vi "Revision Query.vi"(0 "VISA resource name":refnum<visa-resource-name>, 1 "Unit Address (1)":u8=1, 11 "error in (no error)":errorcluster {"code" format="%.0x"}) -> (4 "VISA resource name out":refnum<visa-resource-name>, 8 "Instr Driver Revision":string, 10 "Instr Firmware Revision":string, 15 "error out":errorcluster {"code" format="%.0x"})   [LabVIEW 2010]
doc: "This VI queries the current instrument firmware revision and instrument driver revision.\n\nThis Instrument Driver's Revision number is 1.0.0 and is compatible with Instrument Firmware Revision 7.00\n\nWLF4 Watlow Ramping Controller\nCreated By: Tomas Gres, VSB-TU Ostrava\nRelease Date: 03/2004\nOriginally Developed in LabVIEW Version: 6.1\n\nModification History: \n\nNone"
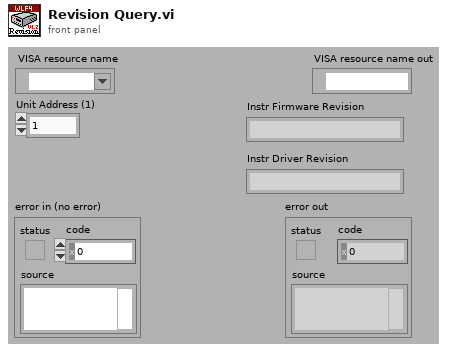
[diagram p1: front panel]
types:
  T1 = enum32{"invalid app kind", "Development System", "Run Time System", "Student Edition", "Embedded LabVIEW", "Evaluation", "Custom"}
  T2 = cluster{"Major":u16, "Minor":u16, "Fix":u16, "Build":u16}
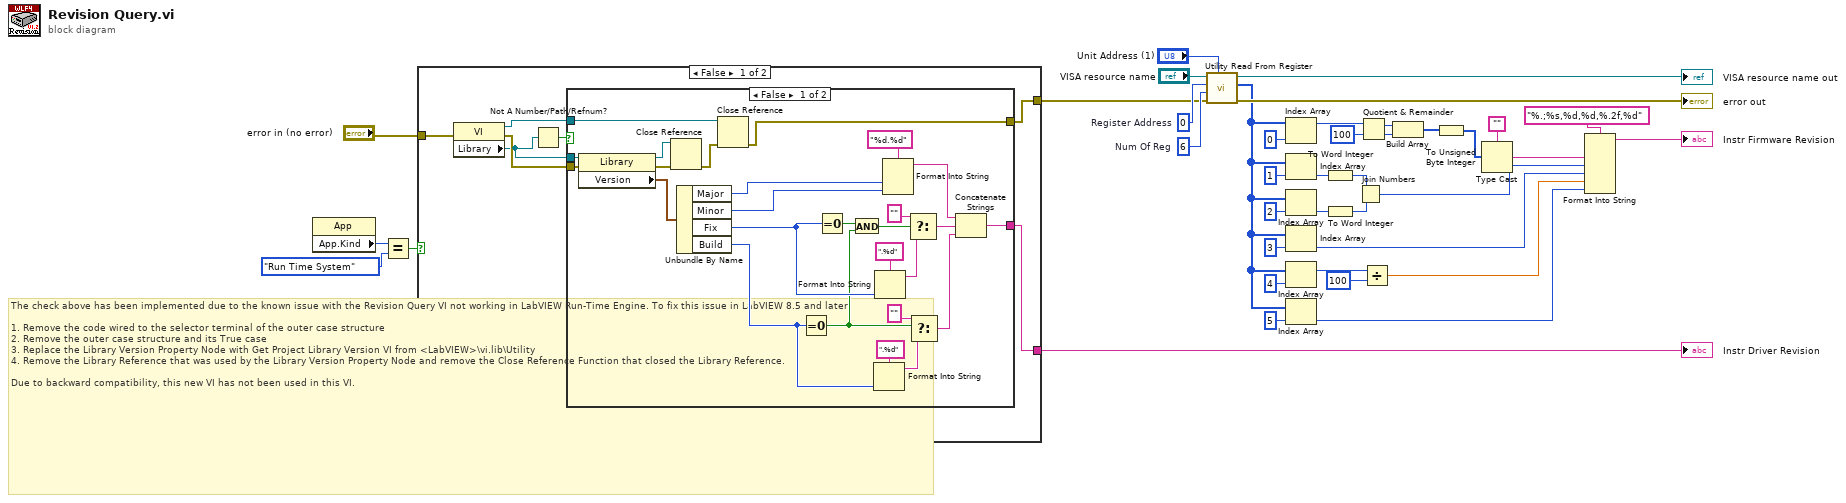
[diagram p0: block diagram]
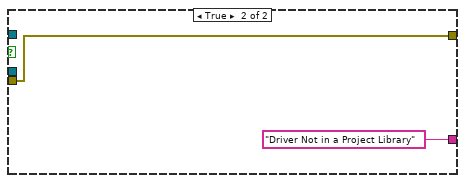
[diagram p2: hidden frame]
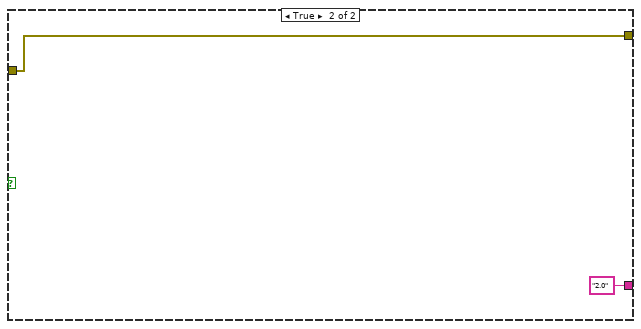
[diagram p3: hidden frame]
diagram:
  w34 = u16 6  # Num Of Reg
  w35 = u16 0  # Register Address
  # "The check above has been implemented due to the known issue with the Revision Query VI not working in LabVIEW Run-Time Engine. To fix this issue in LabVIEW 8.5 and later:\n\n1. Remove the code wired to the selector terminal of the outer case structure\n2. Remove the outer case structure and its True case\n3. Replace the Library Version Property Node with Get Project Library Version VI from <LabVIEW>\\vi.lib\\Utility\n4. Remove the Library Reference that was used by the Library Version Property Node and remove the Close Reference Function that closed the Library Reference.\n\nDue to backward compatibility, this new VI has not been used in this VI."
  n1 = property class="App"() -> ("App.Kind"=w3:T1)  [unwired: 2 in, 2 out]
  n2 = Equal?(x=w3, y=T1."Run Time System") -> (x = y?=w1:bool)
  n3 = case shown="False" w1 {
    tunnel: "error in (no error)" -> [w46 w76]
    tunnel: [w41 "2.0"] -> w5
    tunnel: [w40 w76] -> w4
    frame False {
      n4 = property class="VI"(error in=w46) -> (reference out=w42:refnum<vi>, error out=w45:errorcluster, "Library"=w44:refnum<vi>)  [unwired: 1 in]
      n5 = Not A Number/Path/Refnum?(number/path/refnum=w44) -> (NaN/Path/Refnum?=w43:bool)
      n6 = case shown="False" w43 {
        tunnel: [w51 w73] -> w40
        tunnel: [w50 "Driver Not in a Project Library"] -> w41
        tunnel: w45 -> [w49 w73]
        tunnel: w44 -> [w48 _]
        tunnel: w42 -> [w47 _]
        frame False {
          n7 = property class="Library"(reference=w48, error in=w49) -> (reference out=w71:refnum<vi>, error out=w72:errorcluster, "Version"=w69:T2)
          n8 = Close Reference(reference=w71, error in (no error)=w72) -> (error out=w70:errorcluster)
          n9 = Unbundle By Name(w69) -> ("Major"=w58:u16, "Minor"=w57:u16, "Fix"=w55:u16, "Build"=w56:u16)
          n10 = Close Reference(reference=w47, error in (no error)=w70) -> (error out=w51:errorcluster)
          n11 = Equal To 0?(x=w56) -> (x = 0?=w53:bool)
          n12 = Equal To 0?(x=w55) -> (x = 0?=w54:bool)
          n13 = And(x=w54, y=w53) -> (x .and. y?=w52:bool)
          n14 = Format Into String(format string=".%d", w56) -> (resulting string=w62:string)  [unwired: 2 in, 1 out]
          n15 = Format Into String(format string=".%d", w55) -> (resulting string=w66:string)  [unwired: 2 in, 1 out]
          n16 = Format Into String(format string="%d.%d", w58, w57) -> (resulting string=w64:string)  [unwired: 2 in, 1 out]
          n17 = Select(t="", s=w52, f=w66) -> (s? t:f=w63:string)
          n18 = Select(t="", s=w53, f=w62) -> (s? t:f=w59:string)
          n19 = Concatenate Strings(w64, w63, w59) -> (w50:string)
        }
        frame True {
        }
      }
    }
    frame True {
    }
  }
  "Instr Driver Revision" <- w5
  n20 = call "Utility Read From Register.vi"("Unit Address (1)"="Unit Address (1)", "error in (no error)"=w4, "Num Of Reg (1)"=w34, "Register Address (0)"=w35, "VISA resource name"="VISA resource name") -> ("error out"=→"error out":errorcluster, "Data"=w25:i16[], "VISA resource name out"=→"VISA resource name out":refnum<visa-resource-name>)  [unwired: 4 in]
  n21 = Index Array(array=w25, index=0) -> (element=w22:i16)
  n22 = Index Array(array=w25, index=1) -> (element=w13:i16)
  n23 = Index Array(array=w25, index=2) -> (element=w14:i16)
  n24 = Index Array(array=w25, index=3) -> (element=w9:i16)
  n25 = Index Array(array=w25, index=4) -> (element=w18:i16)
  n26 = Index Array(array=w25, index=5) -> (element=w15:i16)
  n27 = To Word Integer(number=w13) -> (16bit integer=w12:i16)
  n28 = To Word Integer(number=w14) -> (16bit integer=w11:i16)
  n29 = Join Numbers(hi=w12, lo=w11) -> ((hi.lo)=w10:u32)
  n30 = Quotient & Remainder(x=w22, y=i16 100) -> (x-y*floor(x/y)=w20:i16, floor(x/y)=w21:i16)
  n31 = Divide(x=w18, y=i16 100) -> (x/y=w16:dbl)
  n32 = Build Array(w20, w21) -> (w8:i16[])
  n33 = To Unsigned Byte Integer(number=w8) -> (unsigned 8bit integer=w7:u8[])
  n34 = Type Cast(type="", x=w7) -> (*(type *) &x=w24:string)
  n35 = Format Into String(format string="%.;%s,%d,%d,%.2f,%d", w24, w10, w9, w16, w15) -> (resulting string=→"Instr Firmware Revision":string)  [unwired: 2 in, 1 out]
